vi "Entry Console - Create Wash Sequence.vi"(8 "error in (no error)":errorcluster, 11 "Wash Steps":T2) -> (0 "error out":errorcluster, 2 "Wash Sequence":T1[](array[typedef]))   [LabVIEW 2017]
doc: "Transforms Wash Steps cluster to Wash Sequence array."
uses:
  Controls/Entry Console - Wash Steps.ctl
  Controller/Controls/Controller - Wash Step.ctl
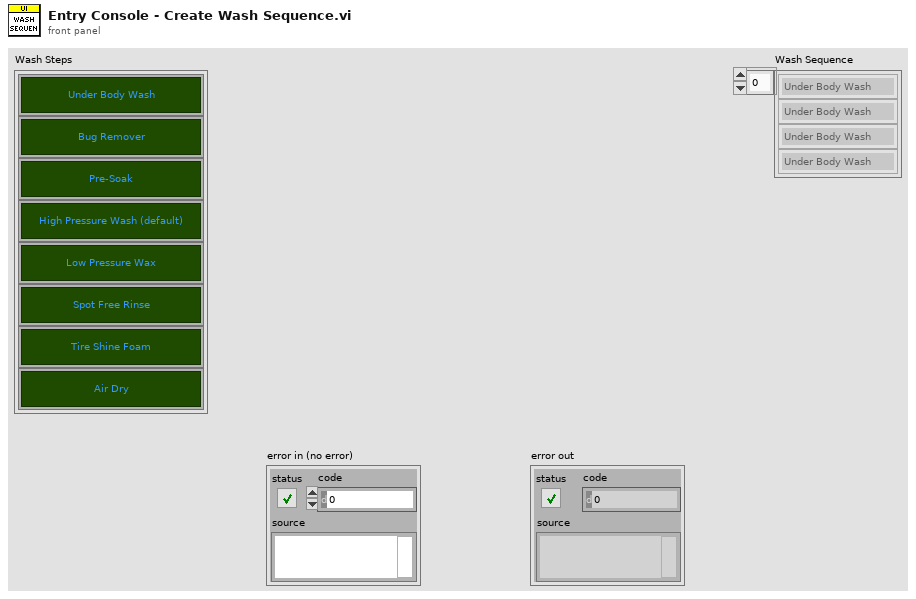
[diagram p1: front panel]
types:
  T1 = typedef "Controller - Wash Step.ctl" = enum16{"Under Body Wash", "Bug Remover", "Pre-Soak", "High Pressure Wash", "Low Pressure Wax", "Spot Free Rinse", "Tire Shine Foam", "Air Dry"}
  T2 = typedef "Entry Console - Wash Steps.ctl" = cluster{"Under Body Wash":bool, "Bug Remover":bool, "Pre-Soak":bool, "High Pressure Wash":bool, "Low Pressure Wax":bool, "Spot Free Rinse":bool, "Tire Shine Foam":bool, "Air Dry":bool}
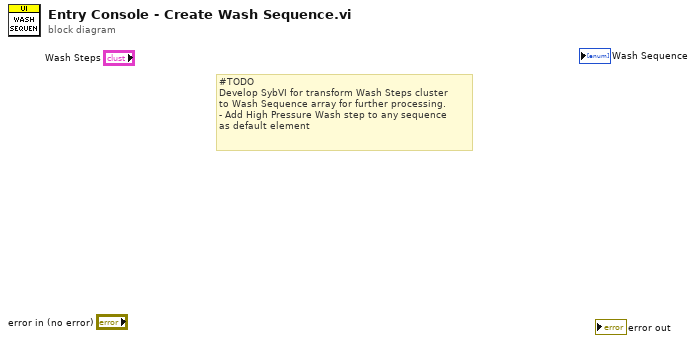
[diagram p0: block diagram]
diagram:
  # "#TODO\nDevelop SybVI for transform Wash Steps cluster\nto Wash Sequence array for further processing.\n- Add High Pressure Wash step to any sequence\nas default element"
